vi "lab8 squence structure.vi"() -> ()   [LabVIEW 2016]
panel:
  out "green":bool
  out "yellow":bool
  out "red":bool
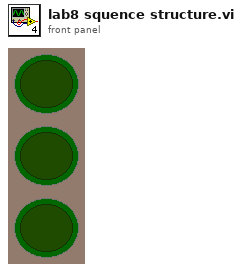
[diagram p1: front panel]
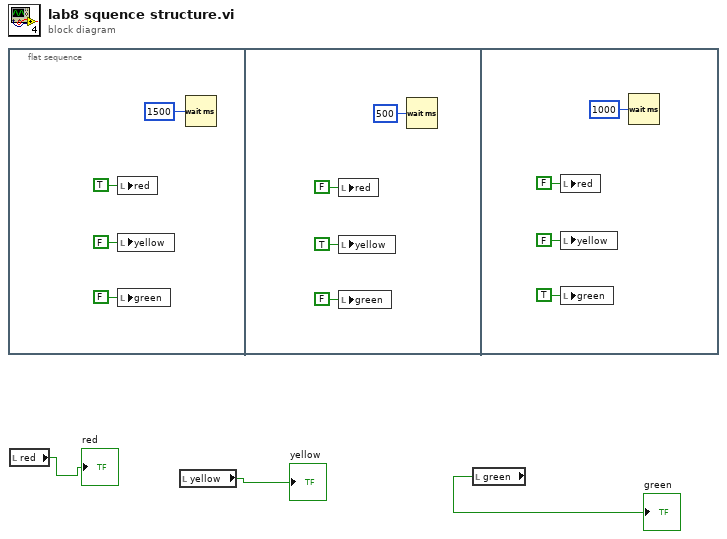
[diagram p0: block diagram]
diagram:
  n1 = flat-sequence {
    frame #0 {
      n2 = local write "red"(TRUE ("red")) -> ()
      n3 = local write "yellow"(FALSE ("yellow")) -> ()
      n4 = local write "green"(FALSE ("green")) -> ()
      n5 = Wait (ms)(milliseconds to wait=u32 1500) -> ()  [unwired: 1 out]
    }
    frame #1 {
      n6 = local write "red"(FALSE ("red")) -> ()
      n7 = local write "yellow"(TRUE ("yellow")) -> ()
      n8 = local write "green"(FALSE ("green")) -> ()
      n9 = Wait (ms)(milliseconds to wait=u32 500) -> ()  [unwired: 1 out]
    }
    frame #2 {
      n10 = local write "red"(FALSE ("red")) -> ()
      n11 = local write "yellow"(FALSE ("yellow")) -> ()
      n12 = local write "green"(TRUE ("green")) -> ()
      n13 = Wait (ms)(milliseconds to wait=u32 1000) -> ()  [unwired: 1 out]
    }
  }
  n14 = local read "red"() -> (→"red":bool)
  n15 = local read "yellow"() -> (→"yellow":bool)
  n16 = local read "green"() -> (→"green":bool)
